vi "Generate Event.vi"(4 "Error In":errorcluster, 7 "Event Data":T2) -> (0 "Error Out":errorcluster)   [LabVIEW 2015, in "Change Source.lvlib"]
uses:
  Change Source.lvlib
  _libraries/Startup Processes/_typedefs/Subpanel Names.ctl
  _typedefs/Event Data.ctl
  _libraries/Startup Processes/Startup Processes.lvlib
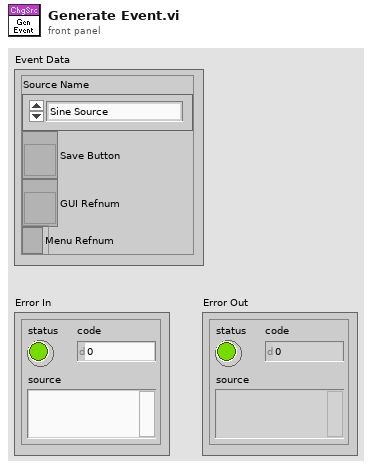
[diagram p1: front panel]
types:
  T1 = typedef "Startup Processes.lvlib/Subpanel Names.ctl" = enum16{"Sine Source", "Ramp Source", "Hen House TC", "Dog House TC", "Out House TC"}
  T2 = cluster{"Source Name":T1, "Save Button":refnum<vi>, "GUI Refnum":refnum<vi>, "Menu Refnum":refnum<k9>}
  T3 = typedef "Change Source.lvlib/Event Data.ctl" = cluster{"Source Name":T1, "Save Button":refnum<vi>, "GUI Refnum":refnum<vi>, "Menu Refnum":refnum<k9>}
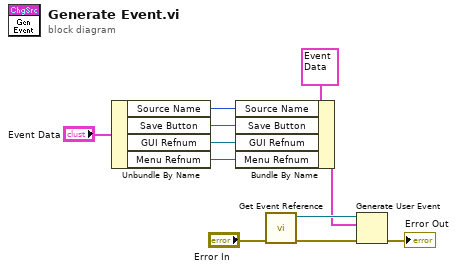
[diagram p0: block diagram]
diagram:
  n1 = Unbundle By Name("Event Data") -> ("Source Name"=w4:T1, "Save Button"=w3:refnum<vi>, "GUI Refnum"=w2:refnum<vi>, "Menu Refnum"=w1:refnum<k9>)
  n2 = Bundle By Name(cluster=T3 {"Source Name"=enum."Sine Source", "Save Button"=refnum, "GUI Refnum"=refnum, "Menu Refnum"=refnum} ("event data"), "Source Name"=w4, "Save Button"=w3, "GUI Refnum"=w2, "Menu Refnum"=w1) -> (w6:T3)
  n3 = call "Get Event Reference.vi"("error in (no error)"="Error In") -> ("error out"=w10:errorcluster, "Change Source"=w9:refnum<user-event>)  [unwired: 5 in]
  n4 = Generate User Event(user event=w9, event data cluster=w6, error in=w10) -> (error out=→"Error Out":errorcluster)  [unwired: 1 in, 1 out]
